vi "Read Initial Cloumn.vi"(8 "error in (no error)":errorcluster, 11 "CCDCamera in":refnum<class "Simulated_CCD_Camera.lvclass">) -> (0 "error out":errorcluster, 2 "Initial Cloumn":u16=1, 3 "CCDCamera out":refnum<class "Simulated_CCD_Camera.lvclass">)   [LabVIEW 2018, in "Simulated_CCD_Camera.lvclass"]
uses:
  Simulated_CCD_Camera.lvclass
  Simulated_CCD_Camera.lvclass/Simulated_CCD_Camera.ctl
  Interface/Interface.lvclass
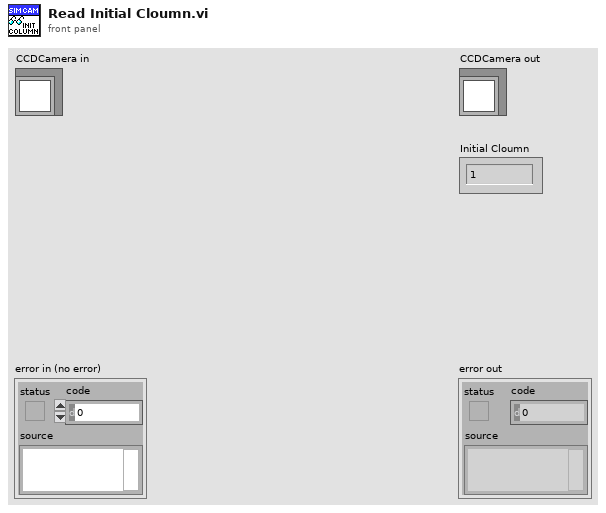
[diagram p1: front panel]
types:
  T1 = cluster{"EXPTIME":sgl, "PREAMP":u8, "READOUT_RATE":u8, "EM_MODE":u8, "EM_GAIN":u16, "BINNING":u16, "INITIAL_LINE":u16, "INITIAL_COLUMN":u16, "FINAL_LINE":u16, "FINAL_COLUMN":u16, "#FRAMES":u32, "SHUTTER_MODE":u8, "COOLER_POWER_STATUS":u16, "TEMP":i8, "#CUBES":u32, "TRIGGER_MODE":u16}
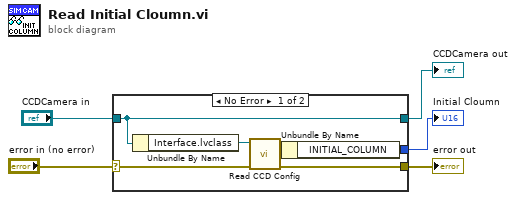
[diagram p0: block diagram]
diagram:
  n1 = case shown="No Error" "error in (no error)" {
    selector: "error in (no error)" -> [w8 w12]
    tunnel: [w9 w12] -> w4
    tunnel: [w7 w13] -> w2
    tunnel: "CCDCamera in" -> [w7 w13]
    tunnel: [w6 _] -> w1
    frame No Error {
      n2 = Unbundle By Name(w7) -> ("Interface.lvclass"=w11:refnum<class "Interface.lvclass">)
      n3 = call "Read CCD Config.vi"("error in (no error)"=w8, "Interface in"=w11) -> ("error out"=w9:errorcluster, "CCD Config"=w10:T1)  [unwired: 7 in, 1 out]
      n4 = Unbundle By Name(w10) -> ("INITIAL_COLUMN"=w6:u16)
    }
    frame Error {
    }
  }
  "error out" <- w4
  "CCDCamera out" <- w2
  "Initial Cloumn" <- w1
